vi "Track 2D.vi"(8 "error in (no error)":errorcluster, 11 "Retiga in":refnum<class "Retiga.lvclass">) -> (0 "error out":errorcluster, 1 "Y move":sgl[unit], 2 "X move":sgl[unit], 3 "Retiga out":refnum<class "Retiga.lvclass">, 5 "move in XY?":bool)   [LabVIEW 2012, in "Retiga.lvclass"]
uses:
  Retiga.lvclass
  Retiga.lvclass/Retiga.ctl
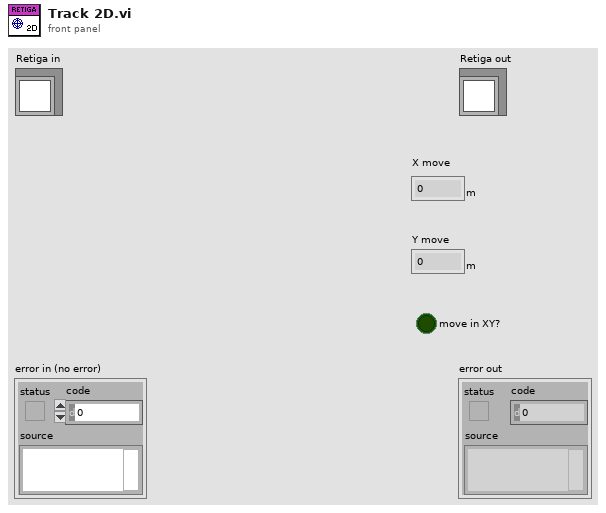
[diagram p1: front panel]
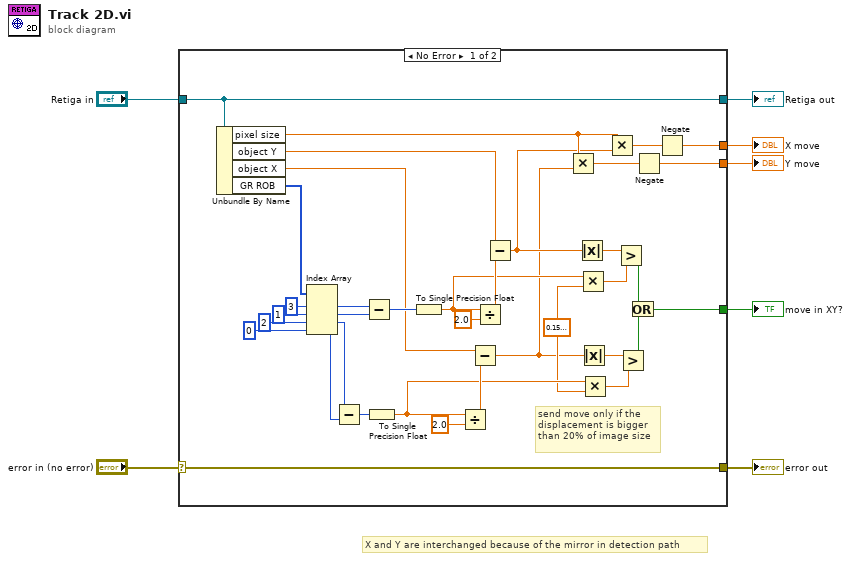
[diagram p0: block diagram]
diagram:
  # "X and Y are interchanged because of the mirror in detection path"
  n1 = case shown="No Error" "error in (no error)" {
    selector: "error in (no error)" -> [w10 w45]
    tunnel: [w10 w45] -> w6
    tunnel: [w11 w44] -> w4
    tunnel: "Retiga in" -> [w11 w44]
    tunnel: [w19 _] -> w1
    tunnel: [w13 _] -> w3
    tunnel: [w12 _] -> w2
    frame No Error {
      w22 = sgl 0.15 ("y")
      # "send move only if the\ndisplacement is bigger\nthan 20% of image size"
      n2 = Unbundle By Name(w11) -> ("pixel size"=w17:sgl[unit], "object Y"=w18:sgl, "object X"=w16:sgl, "GR ROB"=w43:i32[])
      n3 = Index Array(array=w43, index #1=3 ("index"), index #2=1 ("index"), index #3=2 ("index"), index #4=0 ("index")) -> (element #1=w38:i32, element #2=w37:i32, element #3=w24:i32, element #4=w23:i32)
      n4 = Subtract(x=w24, y=w23) -> (x-y=w30:i32)
      n5 = Subtract(x=w38, y=w37) -> (x-y=w36:i32)
      n6 = To Single Precision Float(number=w30) -> (single precision float=w26:sgl)
      n7 = To Single Precision Float(number=w36) -> (single precision float=w32:sgl)
      n8 = Divide(x=w26, y=sgl 2.0) -> (x/y=w28:sgl)
      n9 = Subtract(x=w16, y=w28) -> (x-y=w8:sgl)
      n10 = Divide(x=w32, y=sgl 2.0) -> (x/y=w34:sgl)
      n11 = Subtract(x=w18, y=w34) -> (x-y=w9:sgl)
      n12 = Multiply(x=w17, y=w8) -> (x*y=w14:sgl[unit])
      n13 = Absolute Value(x=w9) -> (abs(x)=w33:sgl)
      n14 = Multiply(x=w32, y=w22) -> (x*y=w31:sgl)
      n15 = Absolute Value(x=w8) -> (abs(x)=w27:sgl)
      n16 = Multiply(x=w26, y=w22) -> (x*y=w25:sgl)
      n17 = Multiply(x=w17, y=w9) -> (x*y=w15:sgl[unit])
      n18 = Greater?(x=w33, y=w31) -> (0:w20:bool)
      n19 = Greater?(x=w27, y=w25) -> (0:w21:bool)
      n20 = Or(x=w20, y=w21) -> (x .or. y?=w19:bool)
      n21 = Negate(x=w14) -> (-x=w12:sgl[unit])
      n22 = Negate(x=w15) -> (-x=w13:sgl[unit])
    }
    frame Error {
    }
  }
  "error out" <- w6
  "Retiga out" <- w4
  "X move" <- w3
  "Y move" <- w2
  "move in XY?" <- w1
